vi "msg_box.vi"(0 "message":string) -> ()   [LabVIEW 2019]
panel:
  in  "Bouton OK":bool
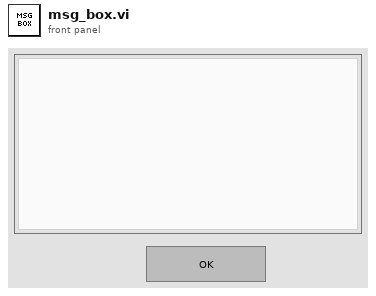
[diagram p1: front panel]
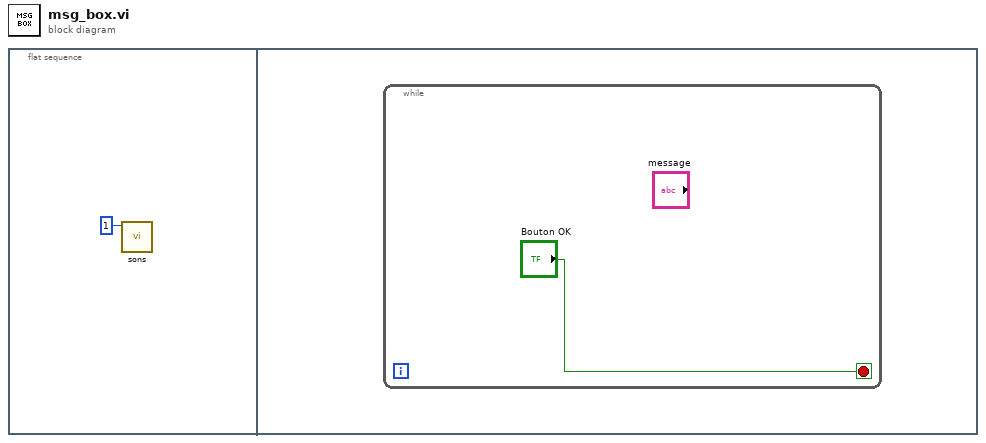
[diagram p0: block diagram]
diagram:
  n1 = flat-sequence {
    frame #0 {
      n2 = call "sons.vi"("Index Son"=i16 1) -> ()  [unwired: 11 in]
    }
    frame #1 {
      n3 = while {
        stop <- "Bouton OK" stop-if-true
      }
    }
  }
